vi "Actor Core.vi"(8 "error in":errorcluster, 11 "Simple Chat in":refnum<class "Simple Chat.lvclass">) -> (0 "error out":errorcluster, 3 "Actor out":refnum<class "Actor.lvclass">)   [LabVIEW 2020, in "Simple Chat.lvlib" / "Simple Chat.lvclass"]
doc: "(<B>Filename</B>: Actor Framework.lvlib:Actor.lvclass:Actor Core.vi)\n\nReceives messages to the actor, reacts to them, and initiates any error handling that may shut the actor down.\n\nDescendant classes may override this VI to append parallel tasks for the actor to complete while it handles messages. Overrides use the Call Parent Class Method node."
uses:
  Simple Chat.lvclass
  C:/Program Files/National Instruments/LabVIEW 2020/vi.lib/ActorFramework/Actor/Actor.lvclass
  <vilib>/ActorFramework/Actor/Actor.lvclass
  <vilib>/ActorFramework/Actor/Actor.lvclass/Actor.ctl
  <vilib>/ActorFramework/Message Enqueuer/Message Enqueuer.lvclass/Message Enqueuer.ctl
  Simple Chat.lvclass/Simple Chat.ctl
  Message Reciever Interface/Message Receiver Interface.lvclass
  Simple Chat Messages/Recieve Message Msg/Receive Message Msg.lvclass/Receive Message Msg.ctl
  <vilib>/ActorFramework/Message Enqueuer/Init from Existing Queue.vi
  <vilib>/ActorFramework/Message Enqueuer/Enqueue.vi
  Simple Chat Messages/Recieve Message Msg/Receive Message Msg.lvclass
  C:/Program Files/National Instruments/LabVIEW 2020/vi.lib/ActorFramework/Message/Message.lvclass
  <vilib>/ActorFramework/Stop Msg/Stop Msg.lvclass
  Actor Pub Sub Channels/Helpers/Get Class Topic Enqueuer.vi
  <vilib>/ActorFramework/Message Priority Queue/Priority Enqueue.vi
  Actor Pub Sub Channels/Helpers/Unsubscribe Topic.vi
  <vilib>/ActorFramework/Message Enqueuer/Message Enqueuer.lvclass
  Actor Pub Sub Channels/Actor Pub Sub Channels.lvlib
panel:
  out "Messages":string
  in  "Message":string
  in  "Send Btn":bool
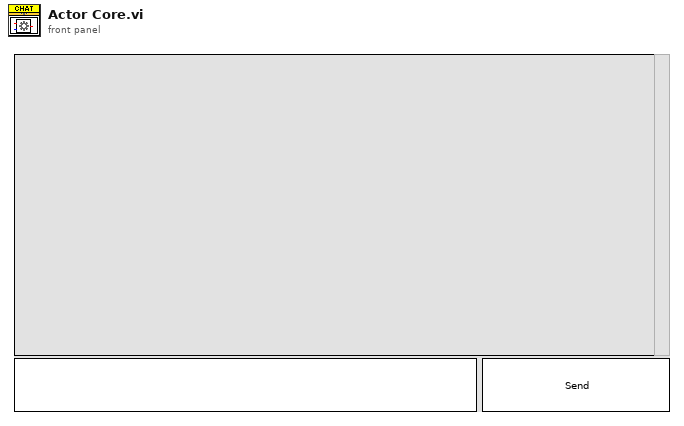
[diagram p1: front panel]
types:
  T1 = enum32{"Invalid", "Standard", "Closed", "Hidden", "Minimized", "Maximized"}
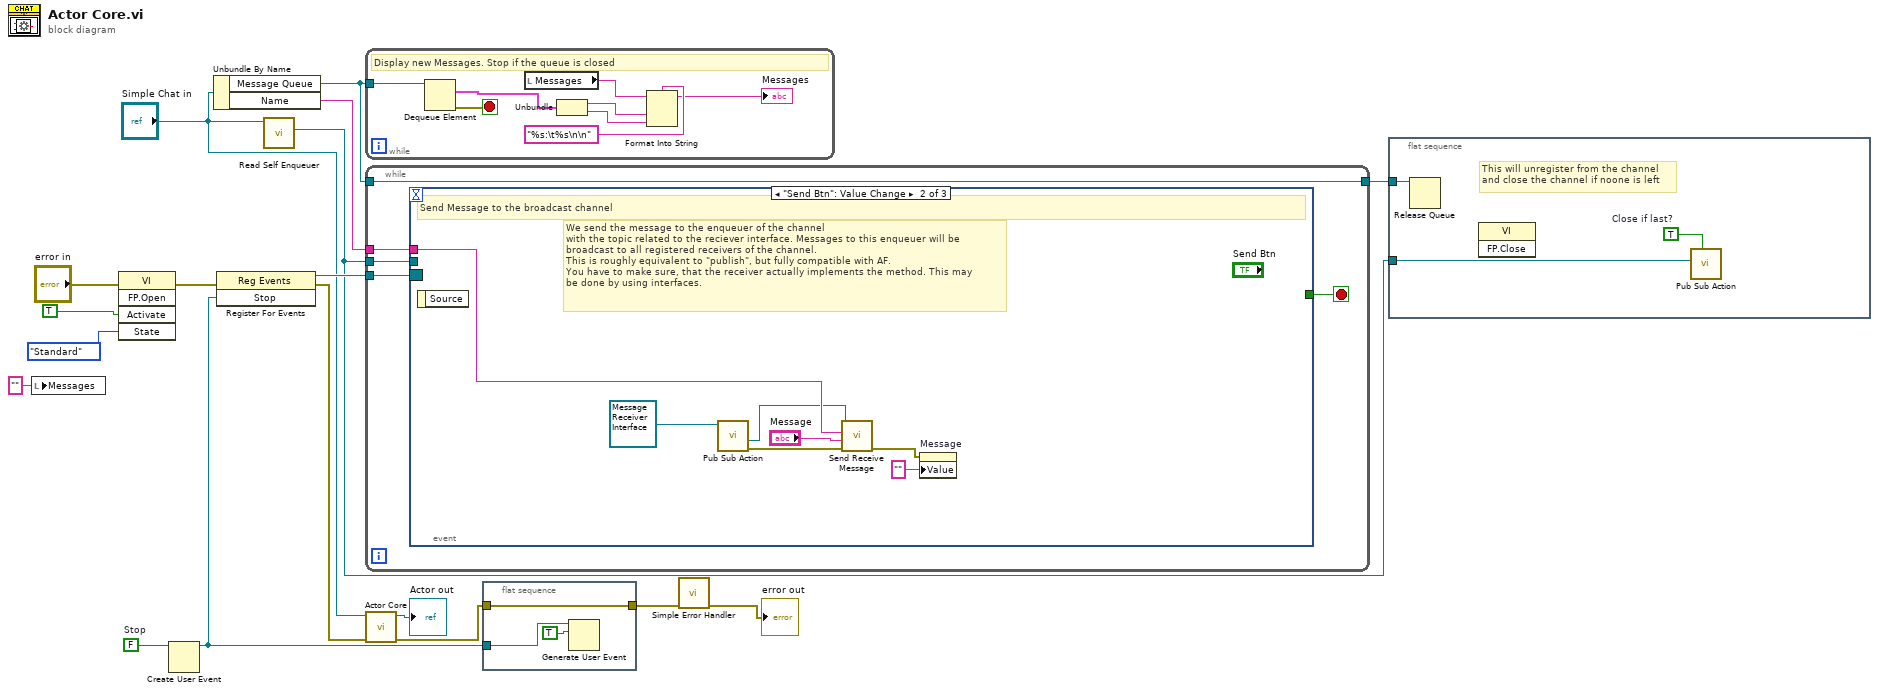
[diagram p0: block diagram]
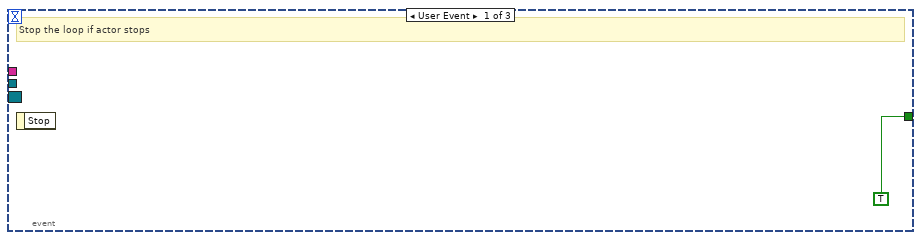
[diagram p2: hidden frame]
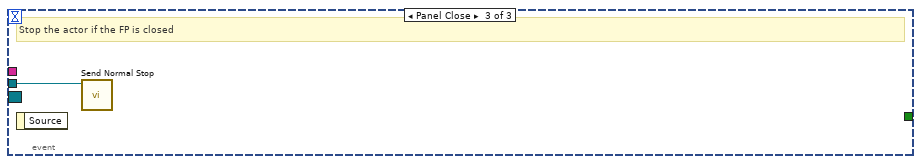
[diagram p3: hidden frame]
diagram:
  w11 = FALSE  # Stop
  n1 = local write "Messages"("" ("Messages")) -> ()
  n2 = invoke class="VI" method="FP.Open"(error in="error in", "Activate"=TRUE ("Activate?"), "State"=T1."Standard") -> (error out=w1:errorcluster)  [unwired: 2 in, 4 out]
  n3 = Create User Event(user event datatype=w11) -> (user event=w10:refnum<user-event>)  [unwired: 1 in, 1 out]
  n4 = Unbundle By Name("Simple Chat in") -> ("Message Queue"=w15:refnum<queue>, "Name"=w16:string)
  n5 = register-events(error in=w1, w10) -> (reference out=w17:refnum<event-registration>, error out=w7:errorcluster)  [unwired: 1 in]
  n6 = call <vilib>:"Read Self Enqueuer.vi"("Actor"="Simple Chat in") -> ("Self Enqueuer"=w13:refnum<class "Message Enqueuer.lvclass">)  [unwired: 10 in]
  n7 = while {
    tunnel: w15 -> [w26]
    stop <- w25 stop-if-true
    # "Display new Messages. Stop if the queue is closed"
    n8 = Dequeue Element(queue=w26) -> (element=w24:cluster{"Sender":string, "Message":string}, error out=w25:errorcluster)  [unwired: 2 in, 2 out]
    n9 = local read "Messages"() -> (w20:string)
    n10 = Unbundle(w24) -> ("Sender"=w23:string, "Message"=w22:string)
    n11 = Format Into String(format string="%s:\t%s\n\n", initial string=w20, w23, w22) -> (resulting string=→"Messages":string)  [unwired: 1 in, 1 out]
  }
  n12 = while {
    tunnel: w17 -> [w31]
    tunnel: w16 -> [w29]
    tunnel: w15 -> [w28]
    tunnel: [w28] -> w6
    tunnel: w13 -> [w27]
    stop <- w30 stop-if-true
    n13 = event shown="[1] \"Send Btn\": Value Change" {
      selector: w31 -> [_ _ _]
      dyn-events: _ -> [_ _ _]
      timeout: _ -> [_ _ _]
      tunnel: [TRUE _ _] -> w30
      tunnel: w29 -> [_ w39 _]
      tunnel: w27 -> [_ _ w40]
      event User Event {
        # "Stop the loop if actor stops"
        n14 = event-data() -> ()  [unwired: 1 in, 1 out]
      }
      event "Send Btn": Value Change {
        # "We send the message to the enqueuer of the channel \nwith the topic related to the reciever interface. Messages to this enqueuer will be\nbroadcast to all registered receivers of the channel. \nThis is roughly equivalent to \"publish\", but fully compatible with AF.\nYou have to make sure, that the receiver actually implements the method. This may\nbe done by using interfaces."
        # "Send Message to the broadcast channel"
        n15 = event-data() -> ()  [unwired: 1 in, 1 out]
        n16 = call-poly "Pub Sub Action.vi"("Topic"=refnum<class "Message Receiver Interface.lvclass"> refnum ("Simple Chat.lvlib:Message Reciever Interface.lvclass")) -> ("error out"=w33:errorcluster, "Topic Enqueuer"=w34:refnum<class "Message Enqueuer.lvclass">)  [unwired: 7 in, 2 out]
        n17 = call "Send Receive Message.vi"("error in (no error)"=w33, "Message"="Message", "Sender"=w39, "Message Enqueuer"=w34) -> ("error out"=w37:errorcluster)  [unwired: 6 in, 1 out]
        n18 = property on="Message" class="Str"(error in=w37, "Value"="" ("Message")) -> ()  [unwired: 1 in, 2 out]
      }
      event Panel Close {
        # "Stop the actor if the FP is closed"
        n19 = event-data() -> ()  [unwired: 1 in, 1 out]
        n20 = call <vilib>:"Send Normal Stop.vi"("Message Enqueuer"=w40) -> ()  [unwired: 10 in, 1 out]
      }
    }
  }
  n21 = call-parent "Actor Core.vi"("error in"=w7, "Actor in"="Simple Chat in") -> ("error out"=w12:errorcluster, "Actor out"=→"Actor out":refnum<class "Actor.lvclass">)  [unwired: 8 in]
  n22 = flat-sequence {
    tunnel: w12 -> [w41]
    tunnel: w10 -> [w42]
    tunnel: [w41] -> w9
    frame #0 {
      n23 = Generate User Event(user event=w42, event data cluster=TRUE ("event data")) -> ()  [unwired: 2 in, 2 out]
    }
  }
  n24 = call <vilib>:"Simple Error Handler.vi"("error in (no error)"=w9) -> ("error out"=→"error out":errorcluster)  [unwired: 4 in, 4 out]
  n25 = flat-sequence {
    tunnel: w6 -> [w46]
    tunnel: w13 -> [w45]
    frame #0 {
      w44 = TRUE  # Close if last?
      # "This will unregister from the channel\nand close the channel if noone is left"
      n26 = Release Queue(queue=w46) -> ()  [unwired: 2 in, 3 out]
      n27 = invoke class="VI" method="FP.Close"() -> ()  [unwired: 3 in, 3 out]
      n28 = call-poly "Pub Sub Action.vi"("Close if last?"=w44, "Receivers Enqueuer"=w45) -> ()  [unwired: 9 in, 1 out]
    }
  }
